vi "test Disconnect.vi"(8 "error in (no error)":errorcluster, 11 "TestCase in":refnum<class "Test TCP Stream Disconnect.lvclass">) -> (0 "error out":errorcluster, 3 "TestCase out":refnum<class "Test TCP Stream Disconnect.lvclass">)   [LabVIEW 2020, in "Test TCP Stream Disconnect.lvclass"]
uses:
  Test TCP Stream Disconnect.lvclass
  <vilib>/addons/_JKI Toolkits/VI Tester/TestCase.llb/TestCase.lvclass
  Source/Protocols/TCP Strategy/TCP Stream Initiator/TCP Stream Initiator.lvclass
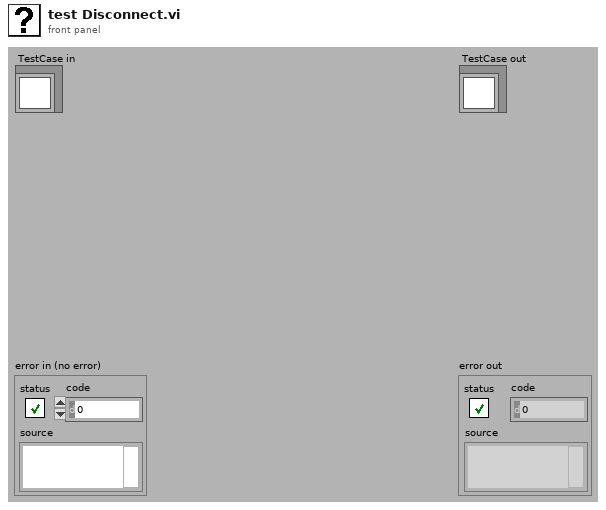
[diagram p1: front panel]
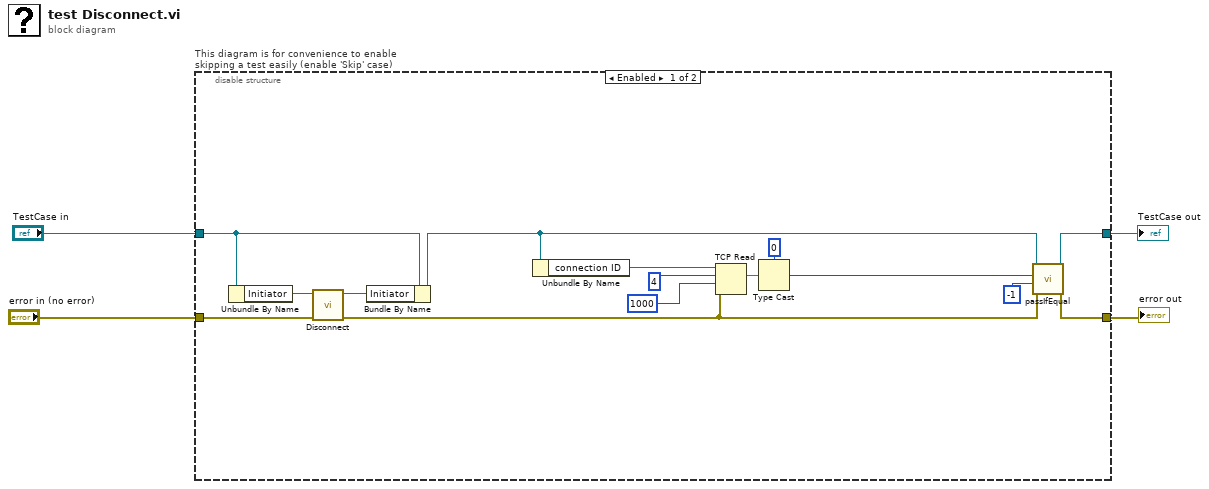
[diagram p0: block diagram]
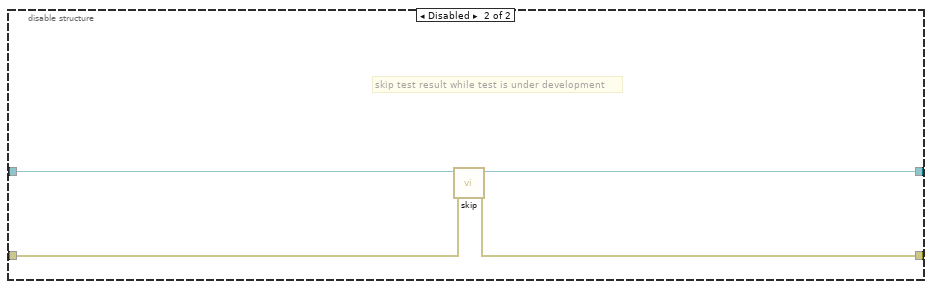
[diagram p2: hidden frame]
diagram:
  n1 = disable-structure "This diagram is for convenience to enable skipping a test easily (enable 'Skip' case)" shown="Enabled" {
    disable-tunnel: "TestCase in" -> [w15 w23]
    disable-tunnel: [w14 w21] -> w2
    disable-tunnel: "error in (no error)" -> [w16 w20]
    disable-tunnel: [w13 w22] -> w1
    frame Enabled {
      n2 = Unbundle By Name(w15) -> ("Initiator"=w19:refnum<class "TCP Stream Initiator.lvclass">)
      n3 = call-dynamic "Disconnect.vi"("error in (no error)"=w16, "TCP Stream in"=w19) -> ("error out"=w10:errorcluster, "TCP Stream out"=w18:refnum<class "TCP Stream Initiator.lvclass">)  [unwired: 8 in]
      n4 = Bundle By Name(cluster=w15, "Initiator"=w18) -> (w17:refnum<class "Test TCP Stream Disconnect.lvclass">)
      n5 = Unbundle By Name(w17) -> ("connection ID"=w12:refnum<k5>)
      n6 = TCP Read(connection ID=w12, bytes to read=4, error in (no error)=w10, 9:1000 ("timeout ms (25000)")) -> (data out=w7:string)  [unwired: 1 in, 2 out]
      n7 = Type Cast(type=0 ("bytes to read"), x=w7) -> (*(type *) &x=w6:i32)
      n8 = call-dynamic "passIfEqual.vi"("error in (no error)"=w10, "y"=-1 ("bytes to read"), "x"=w6, "TestCase in"=w17) -> ("error out"=w13:errorcluster, "TestCase out"=w14:refnum<class "Test TCP Stream Disconnect.lvclass">)  [unwired: 6 in]
    }
    frame Disabled {
      # "skip test result while test is under development"
      n9 = call <vilib>:"skip.vi"("error in (no error)"=w20, "TestCase in"=w23) -> ("error out"=w22:errorcluster, "TestCase out"=w21:refnum<class "Test TCP Stream Disconnect.lvclass">)  [unwired: 8 in]
    }
  }
  "error out" <- w1
  "TestCase out" <- w2
